vi "FRCts20_WebMethods_S3Upload2.vi"(8 "error in (no error)":errorcluster, 11 "Team Index":u32) -> (0 "error out":errorcluster, 1 "Bucket":string="parkway_teamavatars", 2 "Object Path":string, 3 "S3 URL":string)   [LabVIEW 2014, in "FRCts20_Backend_Engine.lvlib"]
uses:
  Backend/source/VI Source/FRCts20_Backend_Engine.lvlib
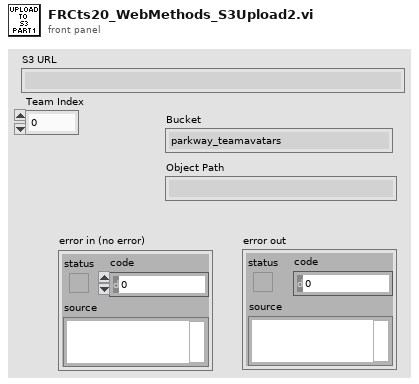
[diagram p1: front panel]
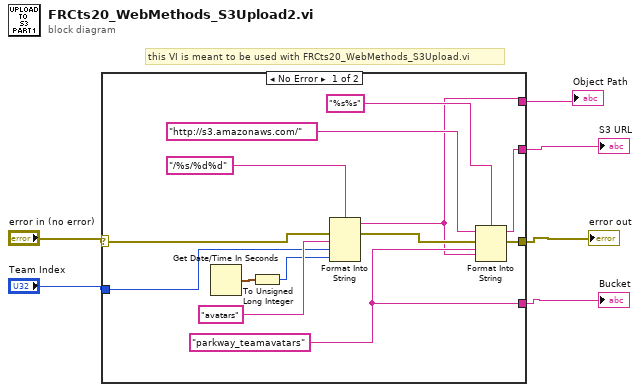
[diagram p0: block diagram]
diagram:
  # "this VI is meant to be used with FRCts20_WebMethods_S3Upload.vi"
  n1 = case shown="No Error" "error in (no error)" {
    selector: "error in (no error)" -> [w8 w20]
    tunnel: [w19 w20] -> w3
    tunnel: [w17 _] -> w2
    tunnel: [w13 _] -> w4
    tunnel: [w12 _] -> w1
    tunnel: "Team Index" -> [w7 _]
    frame No Error {
      w13 = "parkway_teamavatars" ("Bucket")
      n2 = Get Date/Time In Seconds() -> (seconds since 1Jan1904=w11:timestamp)
      n3 = To Unsigned Long Integer(number=w11) -> (unsigned 32bit integer=w9:u32)
      n4 = Format Into String(format string="/%s/%d%d", error in=w8, "avatars" ("Path"), w7, w9) -> (resulting string=w12:string, error out=w14:errorcluster)  [unwired: 1 in]
      n5 = Format Into String(format string="%s%s", initial string="http://s3.amazonaws.com/" ("value"), error in=w14, w13, w12) -> (resulting string=w17:string, error out=w19:errorcluster)
    }
    frame Error {
    }
  }
  "error out" <- w3
  "S3 URL" <- w2
  "Bucket" <- w4
  "Object Path" <- w1
